vi "修改标签.vi"() -> ()   [LabVIEW 2018]
panel:
  in  "写入":bool
  in  "修改":bool
  out "数组 2":string[](array[string])
  out "数组":string[](array[string])
  in  "VI路径":path
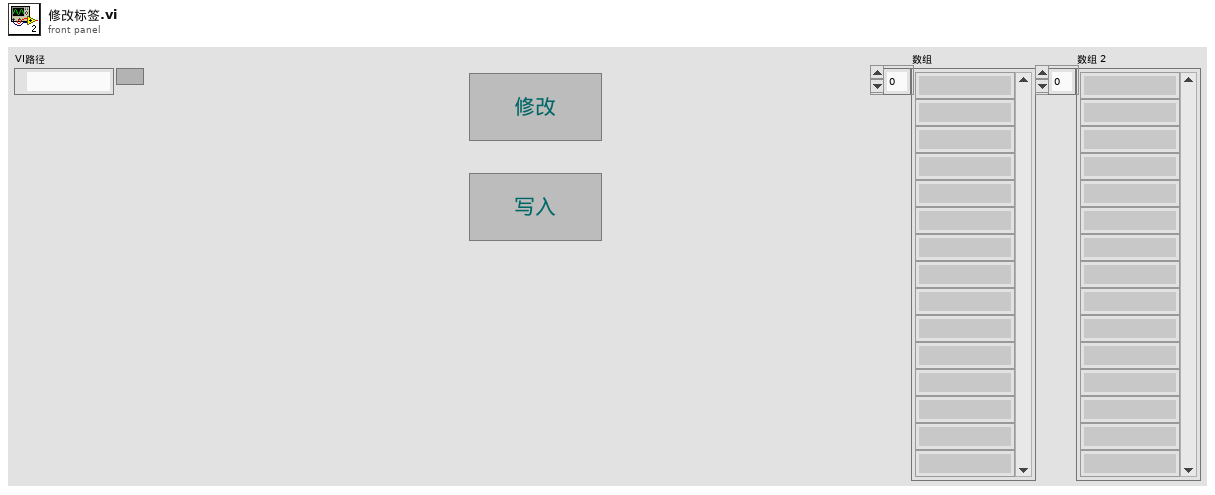
[diagram p1: front panel]
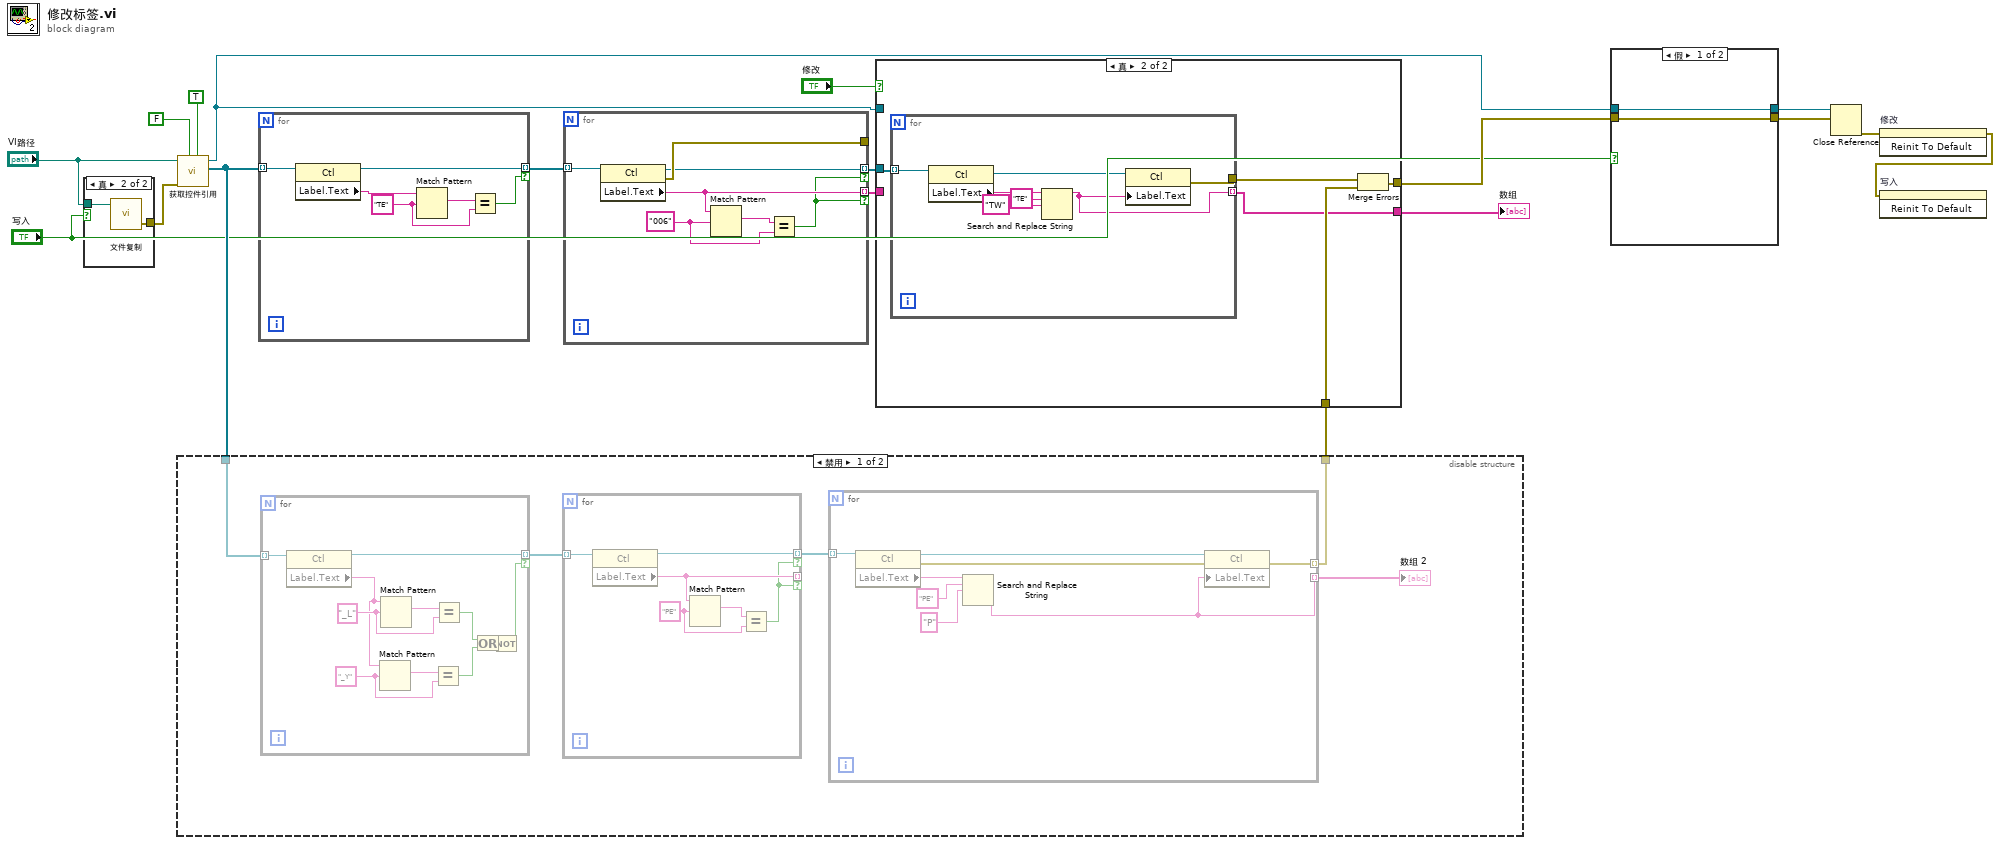
[diagram p0: block diagram]
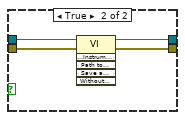
[diagram p4: hidden frame]
diagram:
  n1 = case shown="真" "写入" {
    tunnel: "VI路径" -> [_ w20]
    tunnel: [_ w19] -> w4
    frame False {
    }
    frame True {
      n2 = call "文件复制.vi"("VI路径"=w20) -> ("error out"=w19:errorcluster)  [unwired: 4 in]
    }
  }
  n3 = call "获取控件引用.vi"("以编辑模式打开(T)"=TRUE ("以编辑模式打开"), "布尔(T)"=FALSE, "错误输入（无错误）"=w4, "VI路径"="VI路径") -> ("ContrlRefArray"=w16:refnum<vi>[], "VIRef"=w17:refnum<vi>)  [unwired: 4 in, 1 out]
  n4 = disable-structure shown="禁用" {
    disable-tunnel: w16 -> [w25 _]
    disable-tunnel: [w24 _] -> w14
    frame Disabled {
      n5 = for {
        tunnel: w25 -> [w50] mode=indexing
        tunnel: [w42] -> w23 mode=indexing if=w40
        w46 = "_Y" ("正则表达式")
        w49 = "_L" ("正则表达式")
        n6 = property class="Ctl"(reference=w50) -> (reference out=w42:refnum<vi>, "Label.Text"=w45:string)  [unwired: 1 in, 1 out]
        n7 = Match Pattern(string=w45, regular expression=w46) -> (match substring=w47:string)  [unwired: 1 in, 3 out]
        n8 = Match Pattern(string=w45, regular expression=w49) -> (match substring=w48:string)  [unwired: 1 in, 3 out]
        n9 = Equal?(x=w47, y=w46) -> (x = y?=w43:bool)
        n10 = Equal?(x=w48, y=w49) -> (x = y?=w44:bool)
        n11 = Or(x=w44, y=w43) -> (x .or. y?=w41:bool)
        n12 = Not(x=w41) -> (.not. x?=w40:bool)
      }
      n13 = for {
        tunnel: w23 -> [w39] mode=indexing
        tunnel: [w38] -> _ mode=indexing if=w34
        tunnel: [w35] -> w22 mode=indexing if=w34
        w36 = "PE" ("正则表达式")
        n14 = property class="Ctl"(reference=w39) -> (reference out=w35:refnum<vi>, "Label.Text"=w38:string)  [unwired: 1 in, 1 out]
        n15 = Match Pattern(string=w38, regular expression=w36) -> (match substring=w37:string)  [unwired: 1 in, 3 out]
        n16 = Equal?(x=w37, y=w36) -> (x = y?=w34:bool)
      }
      n17 = for {
        tunnel: w22 -> [w33] mode=indexing
        tunnel: [w26] -> w21 mode=indexing
        tunnel: [w27] -> w24 mode=indexing
        n18 = property class="Ctl"(reference=w33) -> (reference out=w29:refnum<vi>, error out=w28:errorcluster, "Label.Text"=w32:string)  [unwired: 1 in]
        n19 = Search and Replace String(input string=w32, search string="PE" ("正则表达式"), replace string="P" ("正则表达式")) -> (result string=w26:string)  [unwired: 5 in, 3 out]
        n20 = property class="Ctl"(reference=w29, error in=w28, "Label.Text"=w26) -> (error out=w27:errorcluster)  [unwired: 1 out]
      }
      "数组 2" <- w21
    }
    frame Enabled {
    }
  }
  n21 = for {
    tunnel: w16 -> [w56] mode=indexing
    tunnel: [w55] -> w13 mode=indexing if=w54
    w51 = "TE" ("正则表达式")
    n22 = property class="Ctl"(reference=w56) -> (reference out=w55:refnum<vi>, "Label.Text"=w53:string)  [unwired: 1 in, 1 out]
    n23 = Match Pattern(string=w53, regular expression=w51) -> (match substring=w52:string)  [unwired: 1 in, 3 out]
    n24 = Equal?(x=w52, y=w51) -> (x = y?=w54:bool)
  }
  n25 = for {
    tunnel: w13 -> [w63] mode=indexing
    tunnel: [w61] -> w10 mode=indexing if=w57
    tunnel: [w62] -> _
    tunnel: [w58] -> w12 mode=indexing if=w57
    w59 = "006" ("正则表达式")
    n26 = property class="Ctl"(reference=w63) -> (reference out=w58:refnum<vi>, error out=w62:errorcluster, "Label.Text"=w61:string)  [unwired: 1 in]
    n27 = Match Pattern(string=w61, regular expression=w59) -> (match substring=w60:string)  [unwired: 1 in, 3 out]
    n28 = Equal?(x=w60, y=w59) -> (x = y?=w57:bool)
  }
  n29 = case shown="真" "修改" {
    tunnel: w17 -> [_ _]
    tunnel: w14 -> [_ w68]
    tunnel: w12 -> [_ w67]
    tunnel: [w64 w66] -> w11
    tunnel: w10 -> [w64 _]
    tunnel: [_ w65] -> w8
    frame False {
    }
    frame True {
      n30 = for {
        tunnel: w67 -> [w76] mode=indexing
        tunnel: [w70] -> w66 mode=indexing
        tunnel: [w71] -> w69
        n31 = property class="Ctl"(reference=w76) -> (reference out=w72:refnum<vi>, "Label.Text"=w75:string)  [unwired: 1 in, 1 out]
        n32 = Search and Replace String(input string=w75, search string="TE" ("搜索字符串"), replace string="TW" ("替换字符串(\"\")")) -> (result string=w70:string)  [unwired: 5 in, 3 out]
        n33 = property class="Ctl"(reference=w72, "Label.Text"=w70) -> (error out=w71:errorcluster)  [unwired: 1 in, 1 out]
      }
      n34 = Merge Errors(w69, w68) -> (w65:errorcluster)
    }
  }
  "数组" <- w11
  n35 = case shown="假" "写入" {
    tunnel: w17 -> [w78 w82]
    tunnel: w8 -> [w77 w81]
    tunnel: [w78 w80] -> w7
    tunnel: [w77 w79] -> w6
    frame False {
    }
    frame True {
      n36 = invoke class="VI" method="Save.Instrument"(reference=w82, error in=w81) -> (reference out=w80:refnum<vi>, error out=w79:errorcluster)  [unwired: 4 in, 4 out]
    }
  }
  n37 = Close Reference(reference=w7, error in (no error)=w6) -> (error out=w9:errorcluster)
  n38 = invoke on="修改" class="Bool (严格)" method="Reinit To Default"(error in=w9) -> (error out=w5:errorcluster)  [unwired: 2 in, 2 out]
  n39 = invoke on="写入" class="Bool (严格)" method="Reinit To Default"(error in=w5) -> ()  [unwired: 2 in, 3 out]
